vi "FdxCmdEDESubTMDefCvi.vi"(8 "error in":errorcluster, 9 "EDESubTMDefIn":T1, 10 "EDESubscriberHandle":u32, 11 "InstrumentHandle":u32) -> (0 "error out":errorcluster, 3 "InstrumentHandle":u32)   [LabVIEW 2020, in "AIM664LV.lvlib"]
doc: "This function is used to define a Subscriber connection to an EDE Time Manager."
uses:
  AIM664LV.lvlib
  AFDX_LibraryAdmin/FdxGlobalDllPath.vi
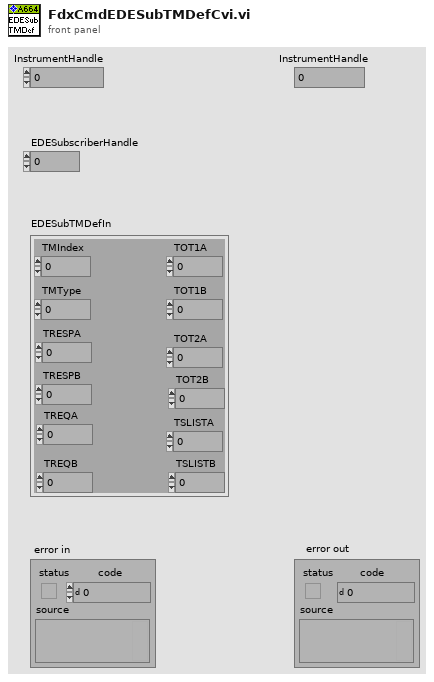
[diagram p1: front panel]
types:
  T1 = cluster{"TMIndex":u32, "TMType":u32, "TRESPA":u32, "TRESPB":u32, "TREQA":u32, "TREQB":u32, "TOT1A":u32, "TOT1B":u32, "TOT2A":u32, "TOT2B":u32, "TSLISTA":u32, "TSLISTB":u32}
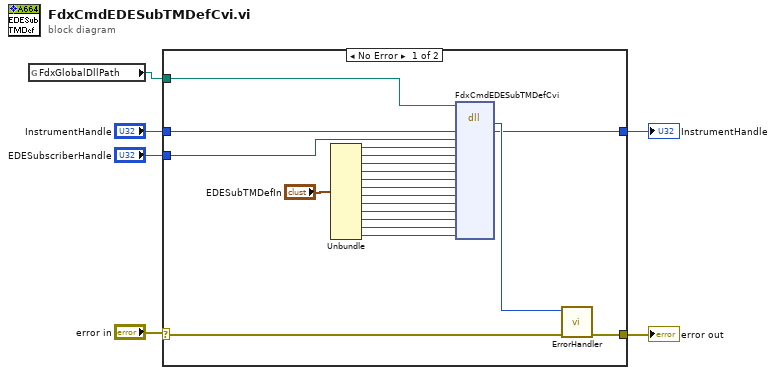
[diagram p0: block diagram]
diagram:
  n1 = global read "FdxGlobalDllPath.vi" "FdxGlobalDllPath"() -> (w4:path)
  n2 = case shown="No Error" "error in" {
    selector: "error in" -> [w25 w28]
    tunnel: [w26 w28] -> w6
    tunnel: w4 -> [w10 _]
    tunnel: [w9 w27] -> w3
    tunnel: "InstrumentHandle" -> [w8 w27]
    tunnel: "EDESubscriberHandle" -> [w7 _]
    frame No Error {
      n3 = Unbundle("EDESubTMDefIn") -> ("TMIndex"=w19:u32, "TMType"=w20:u32, "TRESPA"=w21:u32, "TRESPB"=w22:u32, "TREQA"=w18:u32, "TREQB"=w17:u32, "TOT1A"=w16:u32, "TOT1B"=w15:u32, "TOT2A"=w14:u32, "TOT2B"=w13:u32, "TSLISTA"=w12:u32, "TSLISTB"=w11:u32)
      n4 = dll-call lib="aim_fdx.19.dll" fn="FdxCmdEDESubTMDefCvi"(path in=w10, "InstrumentHandle"=w8, "EDESubscriberHandle"=w7, "TMIndex"=w19, "TMType"=w20, "TRESPA"=w21, "TRESPB"=w22, "TREQA"=w18, "TREQB"=w17, "TOT1A"=w16, "TOT1B"=w15, "TOT2A"=w14, "TOT2B"=w13, "TSLISTA"=w12, "TSLISTB"=w11) -> ("status"=w24:i32, "InstrumentHandle"=w9:u32)  [unwired: 13 in, 4 out]
      n5 = call "ErrorHandler.vi"("error in"=w25, "AIM Error"=w24) -> ("error out"=w26:errorcluster)  [unwired: 9 in]
    }
    frame Error {
    }
  }
  "error out" <- w6
  "InstrumentHandle" <- w3
